vi "Config_privileges.vi"(0 "Enable for None":refnum<vi>[](array[refnum]), 1 "Disable for Default":refnum<vi>[](array[refnum]), 2 "None":T1(ring)=enum."Disabled and Grayed Out", 3 "Log In":bool, 4 "Reinitialize":bool, 5 "error in (no error)":errorcluster, 6 "User":T1(ring)=enum."Disabled and Grayed Out", 8 "Enable for  User":refnum<vi>[](array[refnum]), 9 "Enable for Admin":refnum<vi>[](array[refnum]), 10 "Disable for  User":refnum<vi>[](array[refnum]), 11 "Disable for Admin":refnum<vi>[](array[refnum])) -> (16 "Stop App?":bool, 19 "error out":errorcluster)   [LabVIEW 2012]
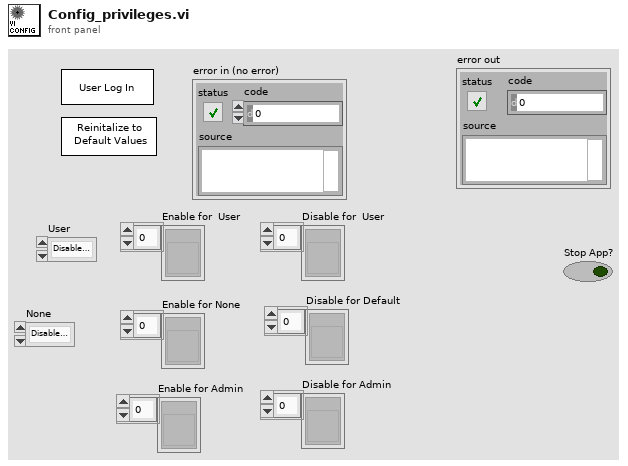
[diagram p1: front panel]
types:
  T1 = enum8{"Enabled", "Disabled", "Disabled and Grayed Out"}
  T2 = typedef "User_Data_Cluster.ctl" = cluster{"Usuario":string, "Password":string, "Account type":T3, "Time Stamp":timestamp}
  T3 = typedef "User Accounts.ctl" = enum16{"None", "User", "Admin"}
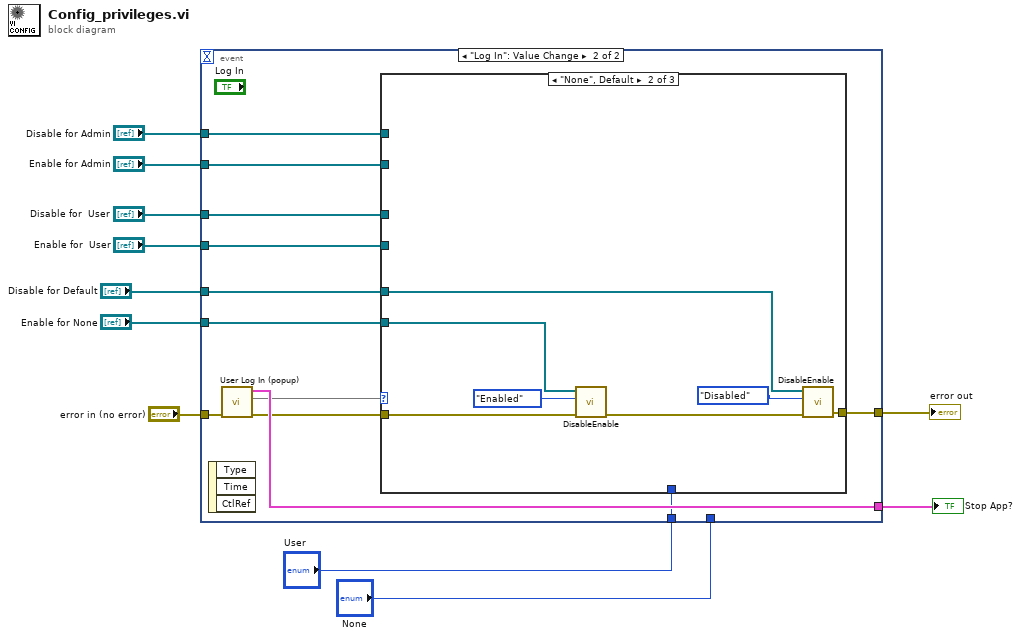
[diagram p0: block diagram]
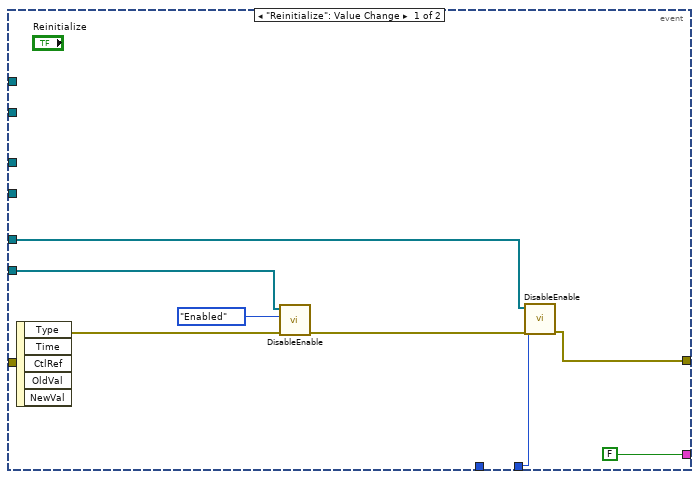
[diagram p2: hidden frame]
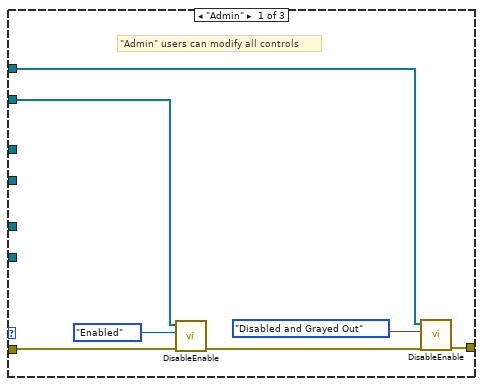
[diagram p3: hidden frame]
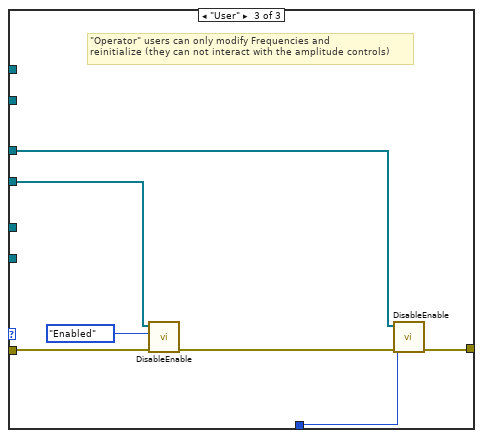
[diagram p4: hidden frame]
diagram:
  n1 = event shown="[1] \"Log In\": Value Change" {
    selector: _ -> [_ _]
    dyn-events: _ -> [_ _]
    timeout: _ -> [_ _]
    tunnel: [FALSE w30] -> w8
    tunnel: "error in (no error)" -> [w15 w31]
    tunnel: [w16 w29] -> w10
    tunnel: "Disable for  User" -> [_ w28]
    tunnel: "Enable for Admin" -> [_ w26]
    tunnel: "Disable for Admin" -> [_ w25]
    tunnel: "Enable for  User" -> [_ w24]
    tunnel: "Disable for Default" -> [w14 w21]
    tunnel: "Enable for None" -> [w13 w20]
    tunnel: "None" -> [w12 _]
    tunnel: "User" -> [_ w23]
    event "Reinitialize": Value Change {
      n2 = event-data() -> ()  [unwired: 1 in, 5 out]
      n3 = call "DisableEnable.vi"("error in (no error)"=w15, 10:T1."Enabled" ("Disabled"), "Array of Control References"=w13) -> ("error out"=w18:errorcluster)  [unwired: 8 in]
      n4 = call "DisableEnable.vi"("error in (no error)"=w18, 10:w12, "Array of Control References"=w14) -> ("error out"=w16:errorcluster)  [unwired: 8 in]
    }
    event "Log In": Value Change {
      n5 = event-data() -> ()  [unwired: 1 in, 3 out]
      n6 = call "User Log In (popup).vi"("error in (no error)"=w31) -> ("error out"=w27:errorcluster, 2:w22, "User-data cluster Out"=w30:T2)  [unwired: 8 in]
      n7 = case shown="\"None\", Default" w22 {
        tunnel: w27 -> [w34 w40 w51]
        tunnel: [w35 w44 w49] -> w29
        tunnel: w28 -> [_ _ w48]
        tunnel: w26 -> [w33 _ _]
        tunnel: w25 -> [w32 _ _]
        tunnel: w24 -> [_ _ w47]
        tunnel: w23 -> [_ _ w46]
        tunnel: w21 -> [_ w43 _]
        tunnel: w20 -> [_ w39 _]
        frame "Admin" {
          # "\"Admin\" users can modify all controls"
          n8 = call "DisableEnable.vi"("error in (no error)"=w34, 10:T1."Enabled" ("Disabled"), "Array of Control References"=w33) -> ("error out"=w38:errorcluster)  [unwired: 8 in]
          n9 = call "DisableEnable.vi"("error in (no error)"=w38, 10:T1."Disabled and Grayed Out" ("Disabled"), "Array of Control References"=w32) -> ("error out"=w35:errorcluster)  [unwired: 8 in]
        }
        frame "None", Default {
          n10 = call "DisableEnable.vi"("error in (no error)"=w40, 10:T1."Enabled" ("Disabled"), "Array of Control References"=w39) -> ("error out"=w41:errorcluster)  [unwired: 8 in]
          n11 = call "DisableEnable.vi"("error in (no error)"=w41, 10:T1."Disabled" ("Disabled"), "Array of Control References"=w43) -> ("error out"=w44:errorcluster)  [unwired: 8 in]
        }
        frame "User" {
          # "\"Operator\" users can only modify Frequencies and \nreinitialize (they can not interact with the amplitude controls)"
          n12 = call "DisableEnable.vi"("error in (no error)"=w51, 10:T1."Enabled" ("Disabled"), "Array of Control References"=w47) -> ("error out"=w52:errorcluster)  [unwired: 8 in]
          n13 = call "DisableEnable.vi"("error in (no error)"=w52, 10:w46, "Array of Control References"=w48) -> ("error out"=w49:errorcluster)  [unwired: 8 in]
        }
      }
    }
  }
  "error out" <- w10
  "Stop App?" <- w8
